vi "while循环的使用(上).vi"() -> ()   [LabVIEW 2018]
panel:
  out "布尔 3":bool
  out "布尔 2":bool
  out "布尔":bool
  # "5.三盏流水灯流水两轮后停止，流水间隔1s"
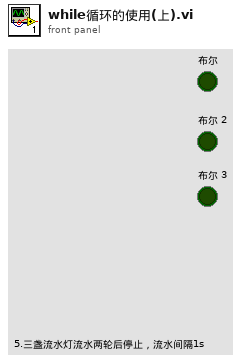
[diagram p1: front panel]
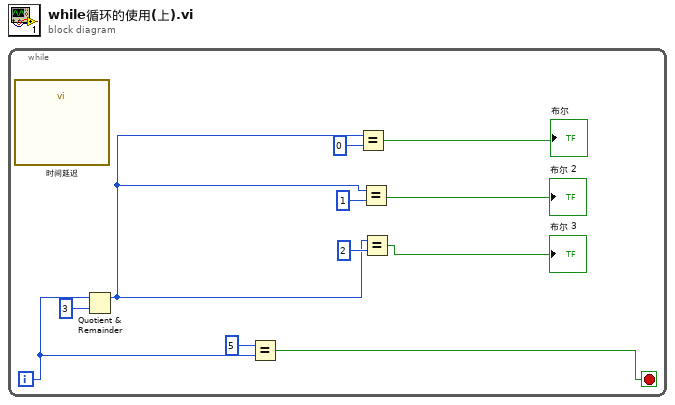
[diagram p0: block diagram]
diagram:
  n1 = while {
    i -> [w3]
    stop <- w1 stop-if-true
    n2 = call "时间延迟"() -> ()  [unwired: 11 in, 1 out]
    n3 = Quotient & Remainder(x=w3, y=3) -> (x-y*floor(x/y)=w6:i32)  [unwired: 1 out]
    n4 = Equal?(x=5, y=w3) -> (x = y?=w1:bool)
    n5 = Equal?(x=w6, y=0) -> (x = y?=→"布尔":bool)
    n6 = Equal?(x=w6, y=1) -> (x = y?=→"布尔 2":bool)
    n7 = Equal?(x=w6, y=2) -> (x = y?=→"布尔 3":bool)
  }
